vi "Count Up U5.vi"(0 "increment":bool=TRUE, 1 "reset":bool) -> (4 "count out":fxp<+,5,5> format="%.21g")   [LabVIEW 2013, in "Engine Simulation Toolkit.lvlib"]
uses:
  Engine Simulation Toolkit.lvlib
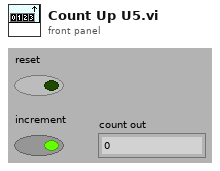
[diagram p1: front panel]
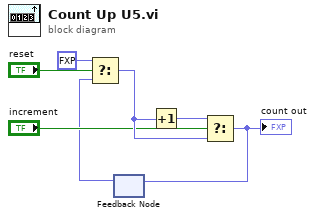
[diagram p0: block diagram]
diagram:
  n1 = feedback #1() -> (w4:fxp<+,5,5>)  [unwired: 1 in]
  n2 = Select(t=fxp<+,5,5> 0.0 ("count in"), s="reset", f=w4) -> (s? t:f=w6:fxp<+,5,5>)
  n3 = Increment(x=w6) -> (x+1=w7:fxp<+,5,5>)
  n4 = Select(t=w7, s="increment", f=w6) -> (s? t:f=w2:fxp<+,5,5>)
  "count out" <- w2
  n5 = feedback-in #1(w2) -> ()
